vi "AlliGator Load Fit Data (Map) mat File v0.1.vi"(8 "Error In":errorcluster, 11 "File Path":path) -> (0 "error out":errorcluster, 1 "Data Description":string, 2 "Decay Fit Options & Parameters":T1={"SYNC Period"=0.0, "Fit Options"={"Show Fit Residuals"=FALSE, "Fit Model"=enum."1-Exponential", "Residual Type"=enum."Standard", "Max Decay Percentile"=0.0, "Min Decay Percentile"=0.0, "Show Full Decay"=FALSE, "Weights"=enum."Unweighted", "Fitting Method"=enum."Least Square", "Compute Parameter Uncertainties"=FALSE, "Periodic Boundaries"=FALSE, "Model Calculation"=enum."Simulation", "Period"=0.0, "Termination Criteria"={"Max Iterations"=0, "Max Function Calls"=0, "Max Time"=0.0, "Function Tolerance"=0.0, "Parameter Tolerance"=0.0, "Gradient Tolerance"=0.0, "Min Lambda"=0.0, "Max Lambda"=0.0, "Initial Tick Count"=0}, "Offset Resolution"=0.0, "Use Local IRF"=FALSE, "Fitting Algorithm"=enum."Levenberg-Marquardt", "Show Confidence Interval "=TRUE, "Confidence Level"=95.0}, "Fit Parameter Constraints"=[], "MLE Baseline Offset"=0.0, "MLE Baseline Offset Type"=enum."Absolute"} {"Fit Options"."Confidence Level" min=0.0 max=100.0; "Fit Options"."Offset Resolution" min=0.0; "Fit Options"."Period" min=0.0; "Fit Options"."Min Decay Percentile" min=0.0 max=1.0; "Fit Options"."Max Decay Percentile" min=0.0 max=100.0; "Fit Parameter Constraints"."Max Value" format="%#.3g"; "Fit Parameter Constraints"."Min Value" format="%#.3g"}, 3 "IRFs & Fit Data Map v3":T13 {"Fit Options: Decay Preprocessing Parameters"."# Folds" min=1}, 4 "[Multiple Decays Fit Parameters SDV]":dbl[][](array[numeric]), 5 "Name":string, 7 "Method":string)   [LabVIEW 2021, in "AlliGator Decay Fit Parameter Map.lvlib"]
doc: "Loads Decay Fit Parameter Map and associated metadata."
uses:
  AlliGator Decay Fit Parameter Map.lvlib
  AlliGator IRFs & Fit Data v3.ctl
  Fits/IRF(X)PSED/Decay Fit Parameters & Derived Quantities List v2.ctl
  Decay Analysis/Decay Preprocessing/AlliGator Decay Preprocessing Parameters.ctl
  Graphs/XY Graph/XY Graph Plot Shift Parameters.ctl
  Graphs/XY Graph/XY Graph Plot Shift Method.ctl
  AlliGator Decay Fit Options & Parameters v4.ctl
  Fits/IRF(X)PSED/Decay Fit Options v4.ctl
  Fits/Decay Convolution/Decay Model.ctl
  Fits/Residual Type.ctl
  Fits/IRF(X)PSED/Fit Weights Type v2.ctl
  Fits/Non-linear Fitting Method v2.ctl
  Fits/Fit Calculation Method.ctl
  Fits/Non-linear Fitting Algorithm.ctl
  Decay Analysis/Decay Fit/AlliGator Decay Fit Parameter Constraints 2.ctl
  Fits/IRF(X)PSED/Decay Fit Parameters In List.ctl
  Fits/IRF(X)PSED/MLE Baseline Offset Type.ctl
  <vilib>/addons/h5labview2/base/lib_path.vi
  <vilib>/addons/h5labview2/base/H5Equery.vi
  <vilib>/addons/h5labview2/dataset/H5Dread.llb/H5Dread.xnode
  <vilib>/addons/h5labview2/file/H5F.lvlib
  <vilib>/addons/h5labview2/group/H5G.lvlib
  Time/Time.lvlib
  Fits/Fits.lvlib
  Strings/Strings.lvlib
  Decay Analysis/Decay Fit/AlliGator Decay Fit.lvlib
  Graphs/XY Graph/XY Graph Add-Ons.lvlib
  Decay Analysis/Decay Preprocessing/AlliGator Decay Preprocessing.lvlib
panel:
  in  "Fit Parameter":T12(ring)
  out "elapsed (relative) seconds":dbl
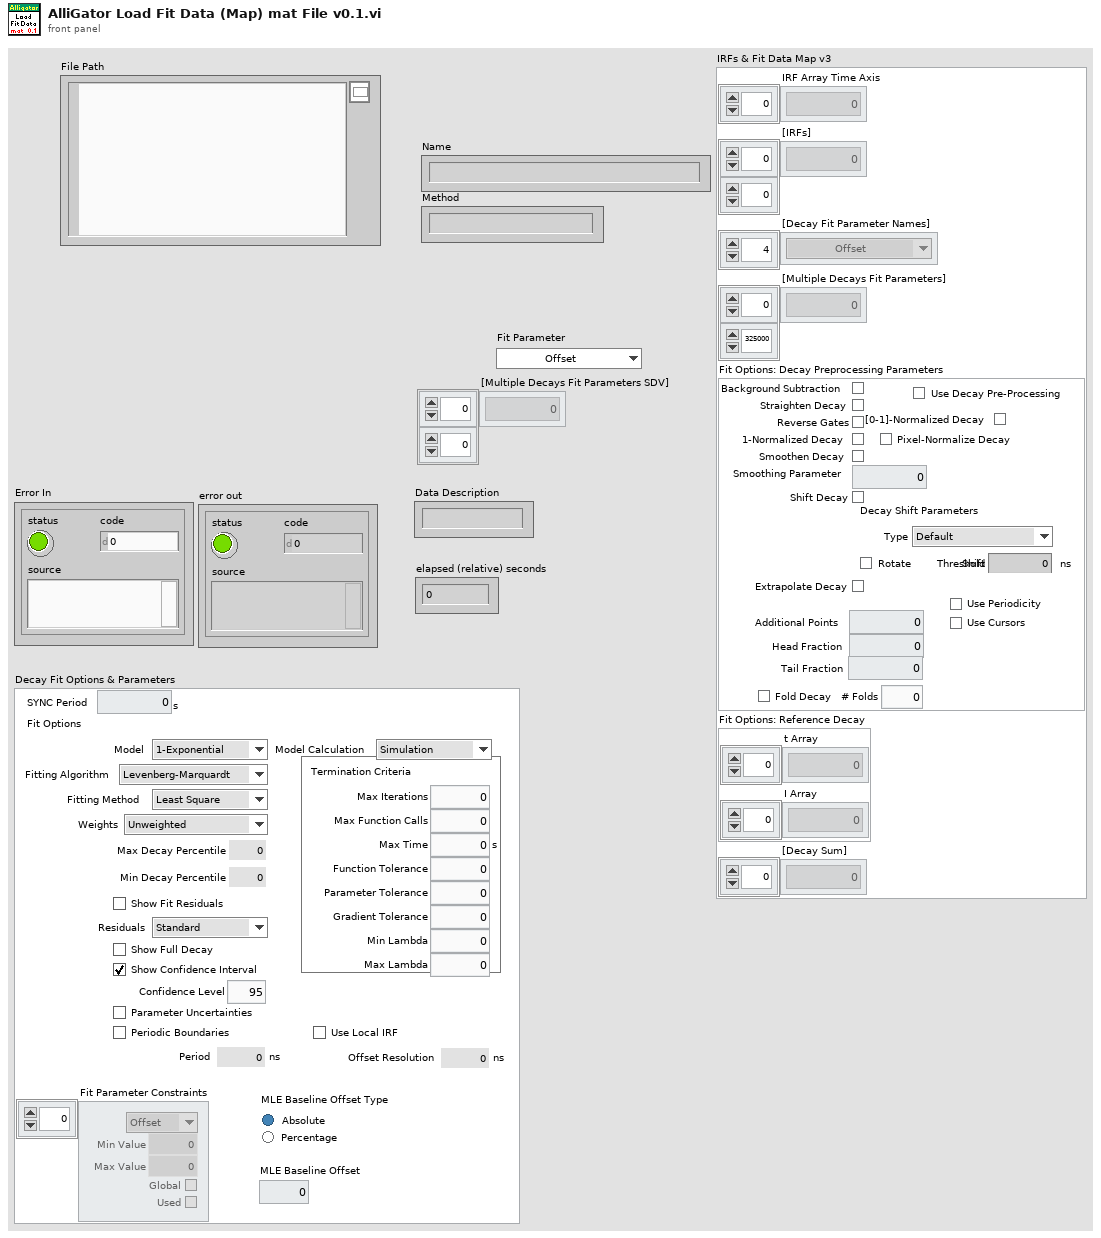
[diagram p1: front panel]
types:
  T1 = typedef "AlliGator Decay Fit Parameter Map.lvlib/AlliGator Decay Fit Options & Parameters v4.ctl" = cluster{"SYNC Period":dbl[unit], "Fit Options":T2, "Fit Parameter Constraints":T9[], "MLE Baseline Offset":dbl, "MLE Baseline Offset Type":T11}
  T2 = typedef "Fits.lvlib/Decay Fit Options v4.ctl" = cluster{"Show Fit Residuals":bool, "Fit Model":T3, "Residual Type":T4, "Max Decay Percentile":dbl, "Min Decay Percentile":dbl, "Show Full Decay":bool, "Weights":T5, "Fitting Method":T6, "Compute Parameter Uncertainties":bool, "Periodic Boundaries":bool, "Model Calculation":T7, "Period":dbl[unit], "Termination Criteria":cluster{"Max Iterations":i32, "Max Function Calls":i32, "Max Time":dbl[unit], "Function Tolerance":dbl, "Parameter Tolerance":dbl, "Gradient Tolerance":dbl, "Min Lambda":dbl, "Max Lambda":dbl, "Initial Tick Count":u32}, "Offset Resolution":dbl[unit], "Use Local IRF":bool, "Fitting Algorithm":T8, "Show Confidence Interval ":bool, "Confidence Level":dbl}
  T3 = typedef "Fits.lvlib/Decay Model.ctl" = enum16{"1-Exponential", "2-Exponentials"}
  T4 = typedef "Fits.lvlib/Residual Type.ctl" = enum16{"Standard", "Normalized", "Reduced"}
  T5 = typedef "Fits.lvlib/Fit Weights Type v2.ctl" = enum16{"Unweighted", "1/Variance (Neyman)", "1/Variance (Pearson)", "Best of All"}
  T6 = typedef "Fits.lvlib/Non-linear Fitting Method v2.ctl" = enum16{"Least Square", "Least Absolute Residual", "Bisquare", "MLE", "-", "Best of All"}
  T7 = typedef "Fits.lvlib/Fit Calculation Method.ctl" = enum16{"Simulation", "Convolution", "Integration"}
  T8 = typedef "Fits.lvlib/Non-linear Fitting Algorithm.ctl" = enum16{"Levenberg-Marquardt", "Trust-Region Dogleg"}
  T9 = typedef "AlliGator Decay Fit.lvlib/AlliGator Decay Fit Parameter Constraints 2.ctl" = cluster{"Fit Parameter":T10, "Min Value":dbl, "Max Value":dbl, "Global":bool, "Used":bool}
  T10 = typedef "Fits.lvlib/Decay Fit Parameters In List.ctl" = enum16{"Offset", "Baseline", "A_1", "tau_1", "A_2", "tau_2"}
  T11 = typedef "Fits.lvlib/MLE Baseline Offset Type.ctl" = enum32{"Absolute", "Percentage"}
  T12 = enum16{"Offset", "Baseline", "A_1", "tau_1", "A_2", "tau_2", "<tau>_1", "f1_1", "f2_1", "<tau>_2", "f1_2", "f2_2", "-", "R^2", "Chi^2"}
  T13 = typedef "AlliGator Decay Fit Parameter Map.lvlib/AlliGator IRFs & Fit Data v3.ctl" = cluster{"IRF Array Time Axis":dbl[], "[IRFs]":dbl[][], "[Decay Fit Parameter Names]":T14[], "[Multiple Decays Fit Parameters]":dbl[][], "Fit Options: Decay Preprocessing Parameters":T15, "Fit Options: Reference Decay":cluster{"t Array":dbl[], "I Array":dbl[]}, "[Decay Sum]":dbl[]}
  T14 = typedef "Fits.lvlib/Decay Fit Parameters & Derived Quantities List v2.ctl" = enum16{"Offset", "Baseline", "A_1", "tau_1", "A_2", "tau_2", "<tau>_a", "f1_a", "f2_a", "<tau>_i", "f1_i", "f2_i", "-", "R^2", "Chi^2"}
  T15 = typedef "AlliGator Decay Preprocessing.lvlib/AlliGator Decay Preprocessing Parameters.ctl" = cluster{"Background Subtraction":bool, "Straighten Decay":bool, "Reverse Gates":bool, "1-Normalized Decay":bool, "Smoothen Decay":bool, "Smoothing Parameter":dbl, "Shift Decay":bool, "Decay Shift Parameters":T16, "Extrapolate Decay":bool, "Additional Points":u32, "Head Fraction":dbl, "Pixel-Normalize Decay":bool, "Use Periodicity":bool, "Use Cursors":bool, "Tail Fraction":dbl, "Use Decay Pre-Processing":bool, "Fold Decay":bool, "# Folds":u32, "[0-1]-Normalized Decay":bool}
  T16 = typedef "XY Graph Add-Ons.lvlib/XY Graph Plot Shift Parameters.ctl" = cluster{"Type":T17, "Shift":dbl[unit], "Threshold":dbl, "Rotate":bool}
  T17 = typedef "XY Graph Add-Ons.lvlib/XY Graph Plot Shift Method.ctl" = enum16{"Default", "CFD", "Threshold", "Cross-Correlation"}
  T18 = typedef "hid_t.ctl" = i64
  T19 = cluster{"IRF Array Time Axis":dbl[], "[IRF]":dbl[][], "[Decay Fit Parameter Name]":T14[], "[Multiple Decays Fit Parameters]":dbl[][]}
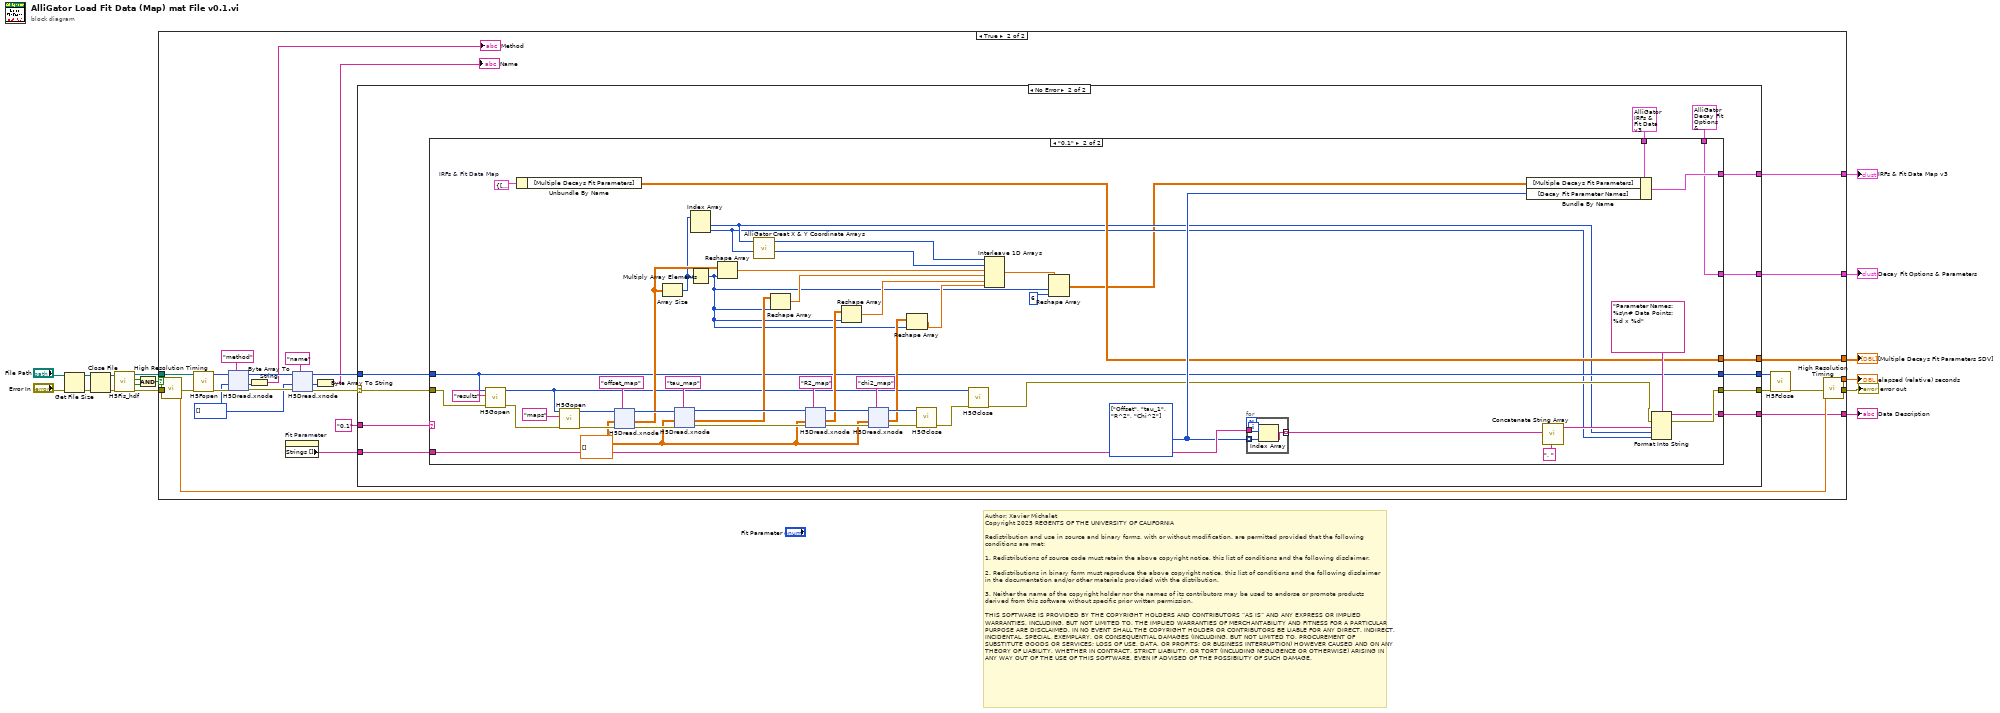
[diagram p0: block diagram]
diagram:
  # "Author: Xavier Michalet\nCopyright 2025 REGENTS OF THE UNIVERSITY OF CALIFORNIA\n\nRedistribution and use in source and binary forms, with or without modification, are permitted provided that the following conditions are met:\n\n1. Redistributions of source code must retain the above copyright notice, this list of conditions and the following disclaimer.\n\n2. Redistributions in binary form must reproduce the above copyright notice, this list of conditions and the following disclaimer in the documentation and/or other materials provided with the distribution.\n\n3. Neither the name of the copyright holder nor the names of its contributors may be used to endorse or promote products derived from this software without specific prior written permission.\n\nTHIS SOFTWARE IS PROVIDED BY THE COPYRIGHT HOLDERS AND CONTRIBUTORS “AS IS” AND ANY EXPRESS OR IMPLIED WARRANTIES, INCLUDING, BUT NOT LIMITED TO, THE IMPLIED WARRANTIES OF MERCHANTABILITY AND FITNESS FOR A PARTICULAR PURPOSE ARE DISCLAIMED. IN NO EVENT SHALL THE COPYRIGHT HOLDER OR CONTRIBUTORS BE LIABLE FOR ANY DIRECT, INDIRECT, INCIDENTAL, SPECIAL, EXEMPLARY, OR CONSEQUENTIAL DAMAGES (INCLUDING, BUT NOT LIMITED TO, PROCUREMENT OF SUBSTITUTE GOODS OR SERVICES; LOSS OF USE, DATA, OR PROFITS; OR BUSINESS INTERRUPTION) HOWEVER CAUSED AND ON ANY THEORY OF LIABILITY, WHETHER IN CONTRACT, STRICT LIABILITY, OR TORT (INCLUDING NEGLIGENCE OR OTHERWISE) ARISING IN ANY WAY OUT OF THE USE OF THIS SOFTWARE, EVEN IF ADVISED OF THE POSSIBILITY OF SUCH DAMAGE."
  n1 = Get File Size(file="File Path", error in="Error In") -> (refnum out=w8:refnum<file>, 0:w9:errorcluster)  [unwired: 1 out]
  n2 = Close File(refnum=w8, error in=w9) -> (path=w7:path, error out=w6:errorcluster)
  n3 = call <vilib>:"H5Fis_hdf.vi"("error in (no error)"=w6, "path in"=w7) -> ("error out"=w13:errorcluster, "valid?"=w16:bool, "exists?"=w17:bool, "path out"=w14:path)  [unwired: 6 in]
  n4 = And(x=w17, y=w16) -> (x .and. y?=w15:bool)
  n5 = case shown="True" w15 {
    tunnel: w14 -> [_ w39]
    tunnel: w13 -> [w18 w46]
    tunnel: [w18 w42] -> w12
    tunnel: [_ w40] -> w5
    tunnel: [_ w38] -> w4
    tunnel: [_ w36] -> w3
    tunnel: [_ w34] -> w2
    tunnel: [_ w33] -> w1
    frame False {
    }
    frame True {
      w24 = u8[] []
      n6 = call "High Resolution Timing.vi"("Error In"=w46) -> ("elapsed (relative) seconds"=w41:dbl, "Error Out"=w43:errorcluster)  [unwired: 16 in, 1 out]
      n7 = call <vilib>:"H5Fopen.vi"("error in (no error)"=w43, "path"=w39) -> ("error out"=w32:errorcluster, "ref out"=w31:T18)  [unwired: 8 in]
      n8 = xnode "H5Dread.xnode"("dataset name (this)"="method", "error in (no error)"=w32, "default"=w24, "ref in"=w31) -> ("error out"=w30:errorcluster, "data"=w23:u8[], "ref out"=w29:i64)  [unwired: 2 in, 1 out]
      n9 = Byte Array To String(unsigned byte array=w23) -> (string=→"Method":string)
      n10 = property on="Fit Parameter" class="Enum (strict)"() -> ("Strings []"=w35:string[])  [unwired: 2 in, 2 out]
      n11 = xnode "H5Dread.xnode"("dataset name (this)"="name", "error in (no error)"=w30, "default"=w24, "ref in"=w29) -> ("error out"=w28:errorcluster, "data"=w21:u8[], "ref out"=w27:i64)  [unwired: 2 in, 1 out]
      n12 = Byte Array To String(unsigned byte array=w21) -> (string=→"Name":string)
      n13 = case shown="No Error" w28 {
        selector: w28 -> [w77 w79]
        tunnel: [w78 w90] -> w45
        tunnel: [w77 w88] -> w44
        tunnel: w27 -> [w78 w89]
        tunnel: "0.1" -> [_ w80]
        tunnel: [_ w87] -> w38
        tunnel: [_ w86] -> w36
        tunnel: w35 -> [_ w85]
        tunnel: [_ w84] -> w34
        tunnel: [_ w83] -> w33
        frame Error {
        }
        frame No Error {
          n14 = case shown="\"0.1\"" w80 {
            tunnel: w89 -> [w92 w102]
            tunnel: [w92 w102] -> w90
            tunnel: [w91 w143] -> w88
            tunnel: [_ w144] -> w87
            tunnel: [_ w142] -> w86
            tunnel: w85 -> [_ w140]
            tunnel: [_ w124] -> w84
            tunnel: [_ w109] -> w83
            tunnel: T13 {"IRF Array Time Axis"=[], "[IRFs]"=[], "[Decay Fit Parameter Names]"=[], "[Multiple Decays Fit Parameters]"=[], "Fit Options: Decay Preprocessing Parameters"={"Background Subtraction"=FALSE, "Straighten Decay"=FALSE, "Reverse Gates"=FALSE, "1-Normalized Decay"=FALSE, "Smoothen Decay"=FALSE, "Smoothing Parameter"=0.0, "Shift Decay"=FALSE, "Decay Shift Parameters"={"Type"=enum."Default", "Shift"=0.0, "Threshold"=0.0, "Rotate"=FALSE}, "Extrapolate Decay"=FALSE, "Additional Points"=0, "Head Fraction"=0.0, "Pixel-Normalize Decay"=FALSE, "Use Periodicity"=FALSE, "Use Cursors"=FALSE, "Tail Fraction"=0.0, "Use Decay Pre-Processing"=FALSE, "Fold Decay"=FALSE, "# Folds"=0, "[0-1]-Normalized Decay"=FALSE}, "Fit Options: Reference Decay"={"t Array"=[], "I Array"=[]}, "[Decay Sum]"=[]} ("IRFs & Fit Data Map") -> [_ w126]
            tunnel: T1 {"SYNC Period"=0.0, "Fit Options"={"Show Fit Residuals"=FALSE, "Fit Model"=enum."1-Exponential", "Residual Type"=enum."Standard", "Max Decay Percentile"=0.0, "Min Decay Percentile"=0.0, "Show Full Decay"=FALSE, "Weights"=enum."Unweighted", "Fitting Method"=enum."Least Square", "Compute Parameter Uncertainties"=FALSE, "Periodic Boundaries"=FALSE, "Model Calculation"=enum."Simulation", "Period"=0.0, "Termination Criteria"={"Max Iterations"=0, "Max Function Calls"=0, "Max Time"=0.0, "Function Tolerance"=0.0, "Parameter Tolerance"=0.0, "Gradient Tolerance"=0.0, "Min Lambda"=0.0, "Max Lambda"=0.0, "Initial Tick Count"=0}, "Offset Resolution"=0.0, "Use Local IRF"=FALSE, "Fitting Algorithm"=enum."Levenberg-Marquardt", "Show Confidence Interval "=TRUE, "Confidence Level"=95.0}, "Fit Parameter Constraints"=[], "MLE Baseline Offset"=0.0, "MLE Baseline Offset Type"=enum."Absolute"} ("Decay Fit Options & Parameters") -> [_ w124]
            tunnel: w79 -> [w91 w108]
            frame "", Default {
            }
            frame "0.1" {
              w118 = dbl[][] [] ("[Multiple Decays Fit Parameters]")
              w125 = T14[] [enum."Offset", enum."tau_1", enum."R^2", enum."Chi^2"] items=["Offset", "Baseline", "A_1", "tau_1", "A_2", "tau_2", "<tau>_a", "f1_a", "f2_a", "<tau>_i", "f1_i", "f2_i", "-", "R^2", "Chi^2"] ("Parameter Name Array")
              w145 = T19 {"IRF Array Time Axis"=[], "[IRF]"=[], "[Decay Fit Parameter Name]"=[], "[Multiple Decays Fit Parameters]"=[]}  # IRFs & Fit Data Map
              n15 = call <vilib>:"H5Gopen.vi"("error in (no error)"=w108, "name"="results" ("dataset name"), "ref in"=w102) -> ("error out"=w106:errorcluster, "group out"=w105:T18)  [unwired: 7 in]
              n16 = Unbundle By Name(w145) -> ("[Multiple Decays Fit Parameters]"=w109:dbl[][])
              n17 = call <vilib>:"H5Gopen.vi"("error in (no error)"=w106, "name"="maps" ("dataset name"), "ref in"=w105) -> ("error out"=w136:errorcluster, "group out"=w135:T18)  [unwired: 7 in]
              n18 = xnode "H5Dread.xnode"("dataset name (this)"="offset_map" ("dataset name"), "error in (no error)"=w136, "default"=w118, "ref in"=w135) -> ("error out"=w134:errorcluster, "data"=w117:dbl[][], "ref out"=w132:i64)  [unwired: 2 in, 1 out]
              n19 = Array Size(array=w117) -> (size(s)=w99:i32[])
              n20 = xnode "H5Dread.xnode"("dataset name (this)"="tau_map" ("dataset name"), "error in (no error)"=w134, "default"=w118, "ref in"=w132) -> ("error out"=w133:errorcluster, "data"=w116:dbl[][], "ref out"=w131:i64)  [unwired: 2 in, 1 out]
              n21 = Index Array(array=w99) -> (element #1=w98:i32, element #2=w97:i32)  [unwired: 2 in]
              n22 = Multiply Array Elements(1:w99) -> (0:w95:i32)
              n23 = Reshape Array(w117, w95) -> (w113:dbl[])
              n24 = call "AlliGator Creat X & Y Coordinate Arrays.vi"("Y"=w97, "X"=w98) -> ("Y Array"=w96:i32[], "X array"=w101:i32[])  [unwired: 8 in]
              n25 = Reshape Array(w116, w95) -> (w112:dbl[])
              n26 = xnode "H5Dread.xnode"("dataset name (this)"="R2_map" ("dataset name"), "error in (no error)"=w133, "default"=w118, "ref in"=w131) -> ("error out"=w123:errorcluster, "data"=w115:dbl[][], "ref out"=w121:i64)  [unwired: 2 in, 1 out]
              n27 = Reshape Array(w115, w95) -> (w111:dbl[])
              n28 = xnode "H5Dread.xnode"("dataset name (this)"="chi2_map" ("dataset name"), "error in (no error)"=w123, "default"=w118, "ref in"=w121) -> ("error out"=w122:errorcluster, "data"=w114:dbl[][], "ref out"=w120:i64)  [unwired: 2 in, 1 out]
              n29 = Reshape Array(w114, w95) -> (w110:dbl[])
              n30 = call <vilib>:"H5Gclose.vi"("error in (no error)"=w122, "group in"=w120) -> ("error out"=w104:errorcluster)  [unwired: 9 in]
              n31 = call <vilib>:"H5Gclose.vi"("error in (no error)"=w104, "group in"=w105) -> ("error out"=w103:errorcluster)  [unwired: 9 in]
              n32 = Interleave 1D Arrays(w101, w96, w113, w112, w111, w110) -> (w100:dbl[])
              n33 = Reshape Array(w100, w95, 6 ("dimension size")) -> (w93:dbl[][])
              n34 = for {
                tunnel: w140 -> [w208]
                tunnel: [w207] -> w139 mode=indexing
                tunnel: w125 -> [w206] mode=indexing
                n35 = Index Array(array=w208, index=w206) -> (element=w207:string)
              }
              n36 = Bundle By Name(cluster=w126, "[Multiple Decays Fit Parameters]"=w93, "[Decay Fit Parameter Names]"=w125) -> (w144:T13)
              n37 = call "Concatenate String Array.vi"("Separator (TAB)"=", ", "String Array"=w139) -> ("Formatted String"=w137:string)  [unwired: 9 in]
              n38 = Format Into String(format string="Parameter Names: %s\n# Data Points: %d x %d", error in=w103, w137, w98, w97) -> (resulting string=w142:string, error out=w143:errorcluster)  [unwired: 1 in]
            }
          }
        }
      }
      n39 = call <vilib>:"H5Fclose.vi"("error in (no error)"=w44, "ref"=w45) -> ("error out"=w37:errorcluster)  [unwired: 9 in]
      n40 = call "High Resolution Timing.vi"("relative seconds (NaN)"=w41, "Error In"=w37) -> ("elapsed (relative) seconds"=w40:dbl, "Error Out"=w42:errorcluster)  [unwired: 15 in, 1 out]
    }
  }
  "error out" <- w12
  "elapsed (relative) seconds" <- w5
  "Data Description" <- w3
  "IRFs & Fit Data Map v3" <- w4
  "Decay Fit Options & Parameters" <- w2
  "[Multiple Decays Fit Parameters SDV]" <- w1
